vi "demoForJoe.TestLauncher.vi"() -> ()   [LabVIEW 2016, in "demoForJoe.lvclass"]
uses:
  demoForJoe.lvclass
  <vilib>/JKI/JKI SMO/SMO/Typedefs/SMOState --Enum.ctl
  C:/Program Files (x86)/National Instruments/LabVIEW 2016/vi.lib/JKI/JKI SMO/SMO/SMO.lvclass
  <vilib>/JKI/JKI SMO/SMO/SMO.lvclass
panel:
  in  "String":string
  out "SMO State":T1
  out "error out":errorcluster
  in  "Stop":bool
  # "Basic SMO Test Launcher"
  # "For instructions on how to use the JKI State Machine Objects, examples and video tutorials, visit:\nhttp://jki.net/state-machine-objects/\n\nJKI State Machine Objects™\nhttp://jki.net/state-machine-objects/\nCopyright (C) 2005-2015, JKI <info@jki.net>\nALL RIGHTS RESERVED"
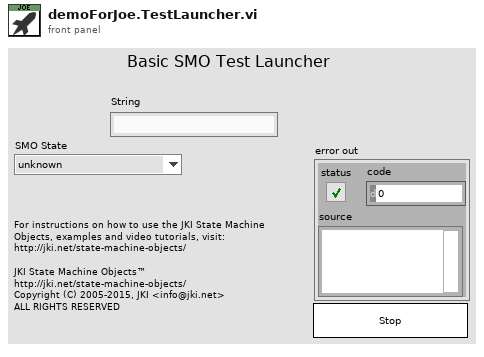
[diagram p1: front panel]
types:
  T1 = typedef "SMO.lvclass/SMOState --Enum.ctl" = enum16{"unknown", "Created", "Started", "Stopped"}
  T2 = typedef "SMO.lvclass/Public Events.ctl" = cluster{"Error":refnum<user-event>, "State":refnum<user-event>, "Reserve State":refnum<user-event>}
  T3 = cluster{"Event Registration Refnum":refnum<event-registration>}
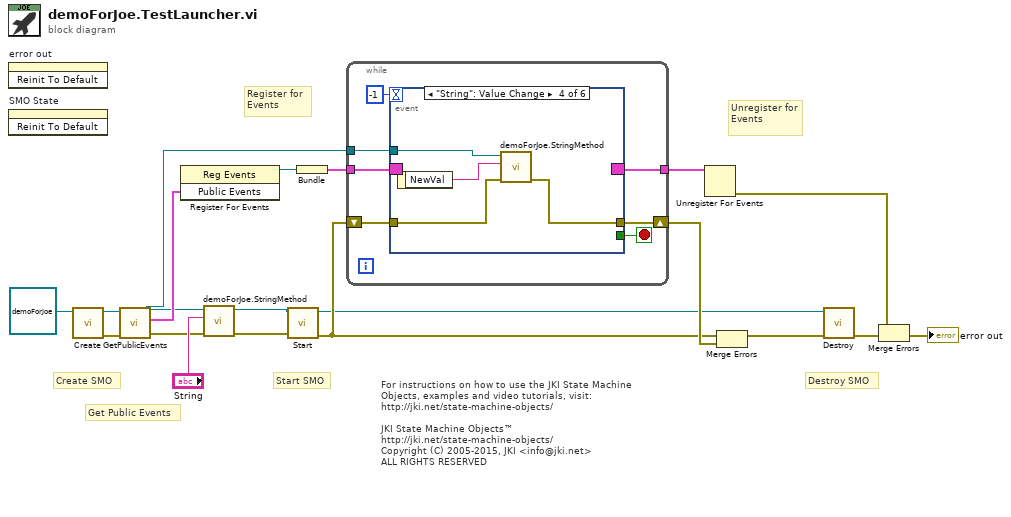
[diagram p0: block diagram]
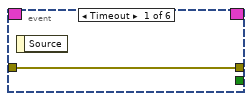
[diagram p2: hidden frame]
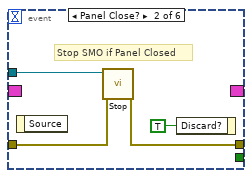
[diagram p3: hidden frame]
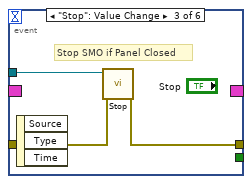
[diagram p4: hidden frame]
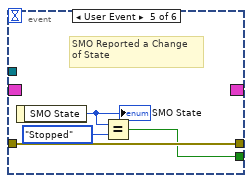
[diagram p5: hidden frame]
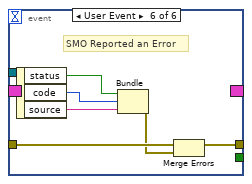
[diagram p6: hidden frame]
diagram:
  # "For instructions on how to use the JKI State Machine Objects, examples and video tutorials, visit:\nhttp://jki.net/state-machine-objects/\n\nJKI State Machine Objects™\nhttp://jki.net/state-machine-objects/\nCopyright (C) 2005-2015, JKI <info@jki.net>\nALL RIGHTS RESERVED"
  # "Get Public Events"
  # "Start SMO"
  # "Destroy SMO"
  # "Create SMO"
  # "Unregister for Events"
  # "Register for Events"
  n1 = invoke on="error out" class="Clust (strict)" method="Reinit To Default"() -> ()  [unwired: 3 in, 3 out]
  n2 = invoke on="SMO State" class="Enum (strict)" method="Reinit To Default"() -> ()  [unwired: 3 in, 3 out]
  n3 = call <vilib>:"Create.vi"("SMO"=refnum<class "demoForJoe.lvclass"> refnum ("SMO.Template.lvclass")) -> ("error out"=w8:errorcluster, "SMO out"=w9:refnum<class "demoForJoe.lvclass">)  [unwired: 8 in, 1 out]
  n4 = call <vilib>:"GetPublicEvents.vi"("error in (no error)"=w8, "SMO"=w9) -> ("error out"=w2:errorcluster, "Public Events"=w7:T2, "SMO out"=w5:refnum<class "demoForJoe.lvclass">)  [unwired: 7 in]
  n5 = register-events(w7) -> (reference out=w6:refnum<event-registration>)  [unwired: 2 in, 1 out]
  n6 = call "demoForJoe.StringMethod.vi"("error in (no error)"=w2, "StringMethod"="String", "demoForJoe"=w5) -> ("error out"=w1:errorcluster, "demoForJoe out"=w4:refnum<class "demoForJoe.lvclass">)  [unwired: 7 in]
  n7 = call <vilib>:"Start.vi"("error in (no error)"=w1, "SMO"=w4) -> ("error out"=w12:errorcluster, "SMO out"=w10:refnum<class "demoForJoe.lvclass">)  [unwired: 8 in]
  n8 = Bundle("Event Registration Refnum"=w6) -> (w18:T3)  [unwired: 1 in]
  n9 = while {
    shift-right: [w25] -> w17
    shift-left: w12 -> [w24]
    tunnel: w18 -> [w23]
    tunnel: [w22] -> w19
    tunnel: w5 -> [w21]
    stop <- w26 stop-if-true
    n10 = event shown="[3] \"String\": Value Change" {
      selector: w23 -> [_ _ _ _ _ _]
      dyn-events: [_ _ _ _ _ _] -> w22
      timeout: -1 -> [_ _ _ _ _ _]
      tunnel: [_ _ _ _ w39 _] -> w26
      tunnel: w21 -> [_ w31 w34 w38 _ _]
      tunnel: [w27 w30 w33 w35 w42 w46] -> w25
      tunnel: w24 -> [w27 w29 w32 w36 w42 w44]
      event Timeout {
        n11 = event-data() -> ()  [unwired: 1 in, 1 out]
      }
      event Panel Close? {
        # "Stop SMO if Panel Closed"
        n12 = event-data() -> ()  [unwired: 1 in, 1 out]
        n13 = call <vilib>:"Stop.vi"("error in (no error)"=w29, "SMO"=w31) -> ("error out"=w30:errorcluster)  [unwired: 8 in, 1 out]
        n14 = event-data("Discard?"=TRUE ("OK")) -> ()  [unwired: 1 in, 1 out]
      }
      event "Stop": Value Change {
        # "Stop SMO if Panel Closed"
        n15 = event-data() -> ()  [unwired: 1 in, 3 out]
        n16 = call <vilib>:"Stop.vi"("error in (no error)"=w32, "SMO"=w34) -> ("error out"=w33:errorcluster)  [unwired: 8 in, 1 out]
      }
      event "String": Value Change {
        n17 = event-data() -> ("NewVal"=w37:string)  [unwired: 1 in]
        n18 = call "demoForJoe.StringMethod.vi"("error in (no error)"=w36, "StringMethod"=w37, "demoForJoe"=w38) -> ("error out"=w35:errorcluster)  [unwired: 7 in, 1 out]
      }
      event User Event {
        # "SMO Reported a Change\nof State"
        n19 = event-data() -> ("SMO State"=w41:T1)  [unwired: 1 in]
        "SMO State" <- w41
        n20 = Equal?(x=w41, y=SMOState_--Enum."Stopped") -> (x = y?=w39:bool)
      }
      event User Event {
        # "SMO Reported an Error"
        n21 = event-data() -> ("status"=w45:bool, "code"=w48:i32, "source"=w47:string)  [unwired: 1 in]
        n22 = Bundle("status"=w45, "code"=w48, "source"=w47) -> (w43:errorcluster)  [unwired: 1 in]
        n23 = Merge Errors(w44, w43) -> (w46:errorcluster)
      }
    }
  }
  n24 = Unregister For Events(event registration refnum=w19) -> (error out=w16:errorcluster)  [unwired: 1 in]
  n25 = Merge Errors(w12, w17) -> (w11:errorcluster)
  n26 = call <vilib>:"Destroy.vi"("error in (no error)"=w11, "SMO"=w10) -> ("error out"=w14:errorcluster)  [unwired: 9 in]
  n27 = Merge Errors(w16, w14) -> (→"error out":errorcluster)
